vi "Perspective Calibration.vi"() -> ()   [LabVIEW 2014]
doc: "Description:\nThis example illustrates the use of a calibration grid to calibrate an image for perspective distortion and converts the locations of features found in the image into the locations in the real world. The example then performs accurate measurements in real world units using these locations.\n\nThis example loads a template image of a grid that is used to calibrate a system, uses the image loaded to learn the calibration from the grid, and measures distances of a distortion template with the learned calibration information."
uses:
  <vilib>/vision/Calibration.llb/Distortion Model.ctl
  <vilib>/vision/Calibration.llb/Distortion Model Types.ctl
  <vilib>/vision/Clamp.llb/Edge Polarity Type.ctl
  <vilib>/vision/Pattern Matching.llb/IMAQ Curve Parameters.ctl
  <vilib>/vision/NI_Vision_Development_Module.lvlib
panel:
  out "Clamp Results":T1(array[cluster])
  in  "Images Tab":T2(tab)
  out "Acquired Image":T3(plugin-control)
  out "Calibration Grid":T3(plugin-control)
  out "Segmented Holes":T3(plugin-control)
  out "Calibration Error Statistics":T4
  # "Overview: Demonstrates how to use a calibration grid to correct for perspective distortion and calculates the real world and pixel distances for parts to illustrate the importance of calibration to make accurate measurements. \nRequirements: Vision Development Software.\nInstructions: Run the VI."
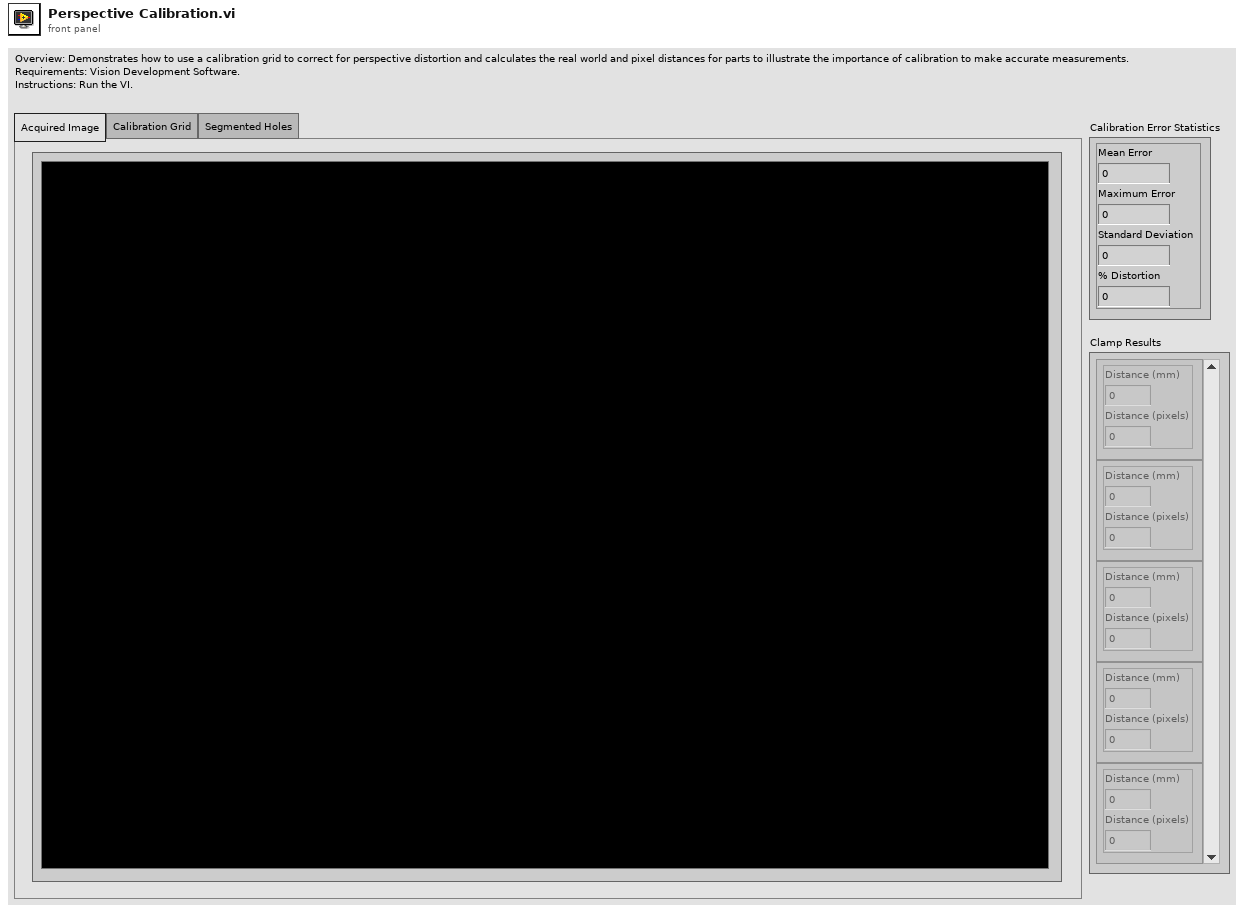
[diagram p1: front panel]
types:
  T1 = cluster{"Distance (mm)":dbl, "Distance (pixels)":dbl}[]
  T2 = enum32{"Acquired Image", "Calibration Grid", "Segmented Holes"}
  T3 = typedef "IMAQ Image.ctl" = refnum<image>
  T4 = cluster{"Mean Error":dbl, "Maximum Error":dbl, "Standard Deviation":dbl, "% Distortion":dbl}
  T5 = typedef "Distortion Model.ctl" = cluster{"Distortion Model":T6, "Polynomial Model Setup":cluster{"Radial Coefficient":u32, "Tangential Coefficients ":bool}}
  T6 = typedef "Distortion Model Types.ctl" = i32
  T7 = typedef "Particle Parameters" = i32
  T8 = cluster{"Measurement Parameter":T7, "Range Lower Value":dbl, "Range Upper Value":dbl, "Range":bool, "Measurement Type":bool}[]
  T9 = typedef "Image Unit" = enum32{"Undefined", "Angström", "Micrometer", "Millimeter", "Centimeter", "Meter", "Kilometer", "Microinch", "Inch", "Feet", "Nautical miles", "Standard miles", "Steps"}
  T10 = typedef "Calibration Reference Points.ctl" = cluster{"Pixel Coordinates":cluster{"X":dbl, "Y":dbl}[], "Real World Coordinates":cluster{"X":dbl, "Y":dbl}[], "Unit":T9, "Image Size":cluster{"X":u32, "Y":u32}}
  T11 = typedef "Error Statistics.ctl" = cluster{"Mean Error":dbl, "Maximum Error":dbl, "Standard Deviation":dbl, "% Distortion":dbl}
  T12 = cluster{"Area":dbl, "Number of Holes":dbl, "Bounding Rect":cluster{"Left":dbl, "Top":dbl, "Right":dbl, "Bottom":dbl}, "Center of Mass":cluster{"X":dbl, "Y":dbl}, "Orientation":dbl, "Dimensions":cluster{"Width":dbl, "Height":dbl}}[]
  T13 = typedef "IMAQ Curve Parameters.ctl" = cluster{"Extraction Mode":u32, "Edge Threshold":i32, "Edge Filter Size":u32, "Min Length":i32, "Row Search Step Size":i32, "Col Search Step Size":i32, "Max Endpoint Gap":i32, "Closed":bool, "Subpixel":bool}
  T14 = cluster{"Show Search Area":bool, "Show Curves":bool, "Show Clamp Locations":bool, "Show Result":bool, "Search Area Color":u32, "Curves Color":u32, "Clamp Locations Color":u32, "Result Color":u32, "Overlay Group Name":string}
  T15 = typedef "Edge Polarity Type.ctl" = u32
  T16 = cluster{"Angle Range (+/-)":dbl, "Edge Polarity":cluster{"Start":T15, "End":T15}}
  T17 = typedef "ROI Descriptor" = cluster{"Global Rectangle":i32[], "Contours":cluster{"ID":enum32{"External", "Internal"}, "Type":u32, "Coordinates":i32[]}[]}
  T18 = cluster{"Distance (Pixels)":dbl, "Distance (Real World)":dbl, "Angle (Absolute)":dbl, "Angle (Relative)":dbl}
  T19 = cluster{"Distance (Real World)":dbl, "Distance (Pixels)":dbl}
  T20 = cluster{"Distance (Real World)":dbl, "Distance (Pixels)":dbl}[]
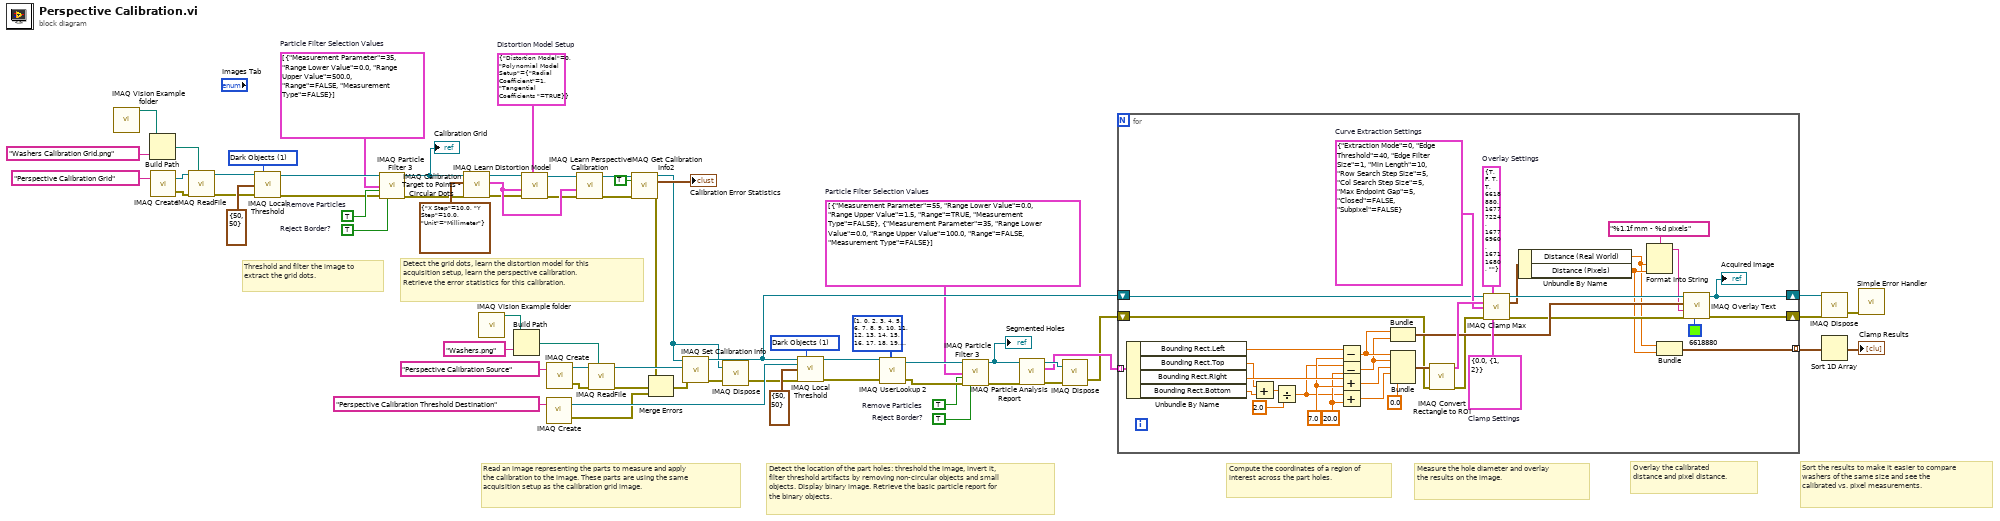
[diagram p0: block diagram]
diagram:
  w28 = TRUE  # Remove Particles
  w29 = TRUE  # Reject Border?
  w39 = T5 {"Distortion Model"=0, "Polynomial Model Setup"={"Radial Coefficient"=1, "Tangential Coefficients "=TRUE}}  # Distortion Model Setup
  w40 = T8 [{"Measurement Parameter"=35, "Range Lower Value"=0.0, "Range Upper Value"=500.0, "Range"=FALSE, "Measurement Type"=FALSE}]  # Particle Filter Selection Values
  w43 = TRUE  # Remove Particles
  w42 = TRUE  # Reject Border?
  w51 = u32 1 items=["Bright Objects", "Dark Objects"] ("Look For (Bright Objects)")
  w53 = T8 [{"Measurement Parameter"=55, "Range Lower Value"=0.0, "Range Upper Value"=1.5, "Range"=TRUE, "Measurement Type"=FALSE}, {"Measurement Parameter"=35, "Range Lower Value"=0.0, "Range Upper Value"=100.0, "Range"=FALSE, "Measurement Type"=FALSE}]  # Particle Filter Selection Values
  w60 = u32 1 items=["Bright Objects", "Dark Objects"] ("Look For (Bright Objects)")
  # "Sort the results to make it easier to compare washers of the same size and see the calibrated vs. pixel measurements."
  # "Overlay the calibrated distance and pixel distance."
  # "Detect the location of the part holes: threshold the image, invert it, filter threshold artifacts by removing non-circular objects and small objects. Display binary image. Retrieve the basic particle report for the binary objects."
  # "Measure the hole diameter and overlay the results on the image."
  # "Compute the coordinates of a region of interest across the part holes."
  # "Read an image representing the parts to measure and apply the calibration to the image. These parts are using the same acquisition setup as the calibration grid image."
  # "Detect the grid dots, learn the distortion model for this acquisition setup, learn the perspective calibration. Retrieve the error statistics for this calibration."
  # "Threshold and filter the image to extract the grid dots."
  n1 = call "IMAQ Vision Example folder.vi"() -> ("Example Image Path"=w26:path)  [unwired: 11 in]
  n2 = Build Path(base path=w26, name or relative path="Washers Calibration Grid.png") -> (appended path=w25:path)
  n3 = call "IMAQ Create"("Image Name"="Perspective Calibration Grid") -> ("New Image"=w64:T3, "error out"=w18:errorcluster)  [unwired: 3 in, 1 out]
  n4 = call "IMAQ ReadFile"("File Path"=w25, "error in (no error)"=w18, "Image"=w64) -> ("error out"=w38:errorcluster, "Image Out"=w21:T3)  [unwired: 2 in, 5 out]
  n5 = call "IMAQ Local Threshold"("Image Src"=w21, "Look For (Bright Objects)"=w51, "Window Size (32x32)"=cluster{"SizeX":i32, "SizeY":i32} {"SizeX"=50, "SizeY"=50}, "error in (no error)"=w38) -> ("Image Dst Out"=w41:T3, "error out"=w37:errorcluster)  [unwired: 4 in, 6 out]
  n6 = call "IMAQ Particle Filter 3"("Image Src"=w41, "Selection Values"=w40, "Keep/Remove Particles (F)"=w43, "error in (no error)"=w37, "Reject Border? (F)"=w42) -> ("Image Dst Out"=w20:T3, "error out"=w36:errorcluster)  [unwired: 4 in, 5 out]
  "Calibration Grid" <- w20
  n7 = call "IMAQ Calibration Target to Points - Circular Dots"("error in (no error)"=w36, "Grid Descriptor"=cluster{"X Step":sgl, "Y Step":sgl, "Unit":T9} {"X Step"=10.0, "Y Step"=10.0, "Unit"=enum."Millimeter"}, "Target Image"=w20) -> ("error out"=w35:errorcluster, "Reference Points"=w48:T10, "Target Image (dup)"=w50:T3)  [unwired: 2 in, 4 out]
  n8 = call "IMAQ Vision Example folder.vi"() -> ("Example Image Path"=w24:path)  [unwired: 11 in]
  n9 = Build Path(base path=w24, name or relative path="Washers.png") -> (appended path=w22:path)
  n10 = call "IMAQ Learn Distortion Model"("Distortion Model Setup"=w39, "error in (no error)"=w35, "Reference Points"=w48, "Calibration Template Image"=w50) -> ("error out"=w34:errorcluster, "Calibration Template Image Out"=w49:T3)  [unwired: 2 in, 4 out]
  n11 = call "IMAQ Create"("Image Name"="Perspective Calibration Threshold Destination") -> ("New Image"=w61:T3, "error out"=w13:errorcluster)  [unwired: 3 in, 1 out]
  n12 = call "IMAQ Create"("Image Name"="Perspective Calibration Source") -> ("New Image"=w63:T3, "error out"=w17:errorcluster)  [unwired: 3 in, 1 out]
  n13 = call "IMAQ Learn Perspective Calibration"("error in (no error)"=w34, "Reference Points"=w48, "Calibration Template Image"=w49) -> ("error out"=w33:errorcluster, "Calibration Template Image Out"=w47:T3)  [unwired: 1 in, 6 out]
  n14 = call "IMAQ ReadFile"("File Path"=w22, "error in (no error)"=w17, "Image"=w63) -> ("error out"=w16:errorcluster, "Image Out"=w56:T3)  [unwired: 2 in, 5 out]
  n15 = call "IMAQ Get Calibration Info2"("Calibration Template Image"=w47, "Return Error Information (False)"=TRUE, "error in (no error)"=w33) -> ("Calibration Template Image (duplicate)"=w3:T3, "Error Statistics"=→"Calibration Error Statistics":T11, "error out"=w15:errorcluster)  [unwired: 10 out]
  n16 = Merge Errors(w15, w16, w13) -> (w14:errorcluster)
  n17 = call "IMAQ Set Calibration Info"("error in (no error)"=w14, "Image Dst"=w56, "Image Src"=w3) -> ("error out"=w4:errorcluster, "Calibrated Image"=w57:T3)  [unwired: 1 in, 6 out]
  n18 = call "IMAQ Dispose"("Image"=w3, "error in (no error)"=w4) -> ("error out"=w2:errorcluster)  [unwired: 4 in]
  n19 = call "IMAQ Local Threshold"("Image Src"=w57, "Look For (Bright Objects)"=w60, "Image Dst"=w61, "Window Size (32x32)"=cluster{"SizeX":i32, "SizeY":i32} {"SizeX"=50, "SizeY"=50}, "error in (no error)"=w2) -> ("Image Dst Out"=w58:T3, "error out"=w32:errorcluster)  [unwired: 3 in, 6 out]
  n20 = call "IMAQ UserLookup 2"("Image Src"=w58, "Lookup Table"=i32[] [1, 0, 2, 3, 4, 5, 6, 7, 8, 9, 10, 11, 12, 13, 14, 15, 16, 17, 18, 19, 20, 21, 22, 23, 24, 25, 26, 27, 28, 29, 30, 31, 32, 33, 34, 35, 36, 37, 38, 39, 40, 41, 42, 43, 44, 45, 46, 47, 48, 49, 50, 51, 52, 53, 54, 55, 56, 57, 58, 59, 60, 61, 62, 63, 64, 65, 66, 67, 68, 69, 70, 71, 72, 73, 74, 75, 76, 77, 78, 79, 80, 81, 82, 83, 84, 85, 86, 87, 88, 89, 90, 91, 92, 93, 94, 95, 96, 97, 98, 99, 100, 101, 102, 103, 104, 105, 106, 107, 108, 109, 110, 111, 112, 113, 114, 115, 116, 117, 118, 119, 120, 121, 122, 123, 124, 125, 126, 127, 128, 129, 130, 131, 132, 133, 134, 135, 136, 137, 138, 139, 140, 141, 142, 143, 144, 145, 146, 147, 148, 149, 150, 151, 152, 153, 154, 155, 156, 157, 158, 159, 160, 161, 162, 163, 164, 165, 166, 167, 168, 169, 170, 171, 172, 173, 174, 175, 176, 177, 178, 179, 180, 181, 182, 183, 184, 185, 186, 187, 188, 189, 190, 191, 192, 193, 194, 195, 196, 197, 198, 199, 200, 201, 202, 203, 204, 205, 206, 207, 208, 209, 210, 211, 212, 213, 214, 215, 216, 217, 218, 219, 220, 221, 222, 223, 224, 225, 226, 227, 228, 229, 230, 231, 232, 233, 234, 235, 236, 237, 238, 239, 240, 241, 242, 243, 244, 245, 246, 247, 248, 249, 250, 251, 252, 253, 254, 255], "error in (no error)"=w32) -> ("Image Dst Out"=w54:T3, "error out"=w31:errorcluster)  [unwired: 2 in, 2 out]
  n21 = call "IMAQ Particle Filter 3"("Image Src"=w54, "Selection Values"=w53, "Keep/Remove Particles (F)"=w28, "error in (no error)"=w31, "Reject Border? (F)"=w29) -> ("Image Dst Out"=w19:T3, "error out"=w30:errorcluster)  [unwired: 4 in, 5 out]
  "Segmented Holes" <- w19
  n22 = call "IMAQ Particle Analysis Report"("error in (no error)"=w30, "Image"=w19) -> ("error out"=w12:errorcluster, "Particle Reports (Pixels)"=w10:T12, "Image Out (duplicate)"=w11:T3)  [unwired: 1 in, 6 out]
  n23 = call "IMAQ Dispose"("Image"=w11, "error in (no error)"=w12) -> ("error out"=w9:errorcluster)  [unwired: 4 in]
  n24 = for {
    tunnel: w10 -> [w101] mode=indexing
    shift-right: [w72] -> w7
    shift-left: w57 -> [w83]
    shift-right: [w74] -> w8
    shift-left: w9 -> [w68]
    tunnel: [w69] -> w6 mode=indexing
    w90 = T13 {"Extraction Mode"=0, "Edge Threshold"=40, "Edge Filter Size"=1, "Min Length"=10, "Row Search Step Size"=5, "Col Search Step Size"=5, "Max Endpoint Gap"=5, "Closed"=FALSE, "Subpixel"=FALSE}  # Curve Extraction Settings
    w88 = T14 {"Show Search Area"=TRUE, "Show Curves"=FALSE, "Show Clamp Locations"=TRUE, "Show Result"=TRUE, "Search Area Color"=6618880, "Curves Color"=16777224, "Clamp Locations Color"=16776960, "Result Color"=16711680, "Overlay Group Name"=""}  # Overlay Settings
    w89 = T16 {"Angle Range (+/-)"=0.0, "Edge Polarity"={"Start"=1, "End"=2}}  # Clamp Settings
    w93 = 20.0 ("y")
    w98 = 7.0 ("y")
    n25 = Unbundle By Name(w101) -> ("Bounding Rect.Left"=w86:dbl, "Bounding Rect.Top"=w77:dbl, "Bounding Rect.Right"=w99:dbl, "Bounding Rect.Bottom"=w76:dbl)
    n26 = Add(x=w77, y=w76) -> (x+y=w95:dbl)
    n27 = Divide(x=w95, y=2.0) -> (x/y=w84:dbl)
    n28 = Subtract(x=w86, y=w98) -> (x-y=w81:dbl)
    n29 = Subtract(x=w84, y=w93) -> (x-y=w80:dbl)
    n30 = Add(x=w99, y=w98) -> (x+y=w97:dbl)
    n31 = Add(x=w84, y=w93) -> (x+y=w96:dbl)
    n32 = Bundle(w81, w80) -> (w79:cluster{dbl, dbl})  [unwired: 1 out]
    n33 = Bundle(w81, w80, w97, w96, "y"=0.0) -> (w100:cluster{dbl, dbl, dbl, dbl, "y":dbl})  [unwired: 1 out]
    n34 = call "IMAQ Convert Rectangle to ROI"("error in (no error)"=w68, "Rectangle"=w100) -> ("error out"=w67:errorcluster, "ROI Descriptor"=w91:T17)  [unwired: 7 out]
    n35 = call "IMAQ Clamp Max"("Source Image"=w83, "Overlay Settings"=w88, "ROI Descriptor"=w91, "Curve Extraction Settings"=w90, "error in (no error)"=w67, "Clamp Settings"=w89) -> ("Image Out"=w82:T3, "Clamp Results"=w75:T18, "error out"=w73:errorcluster)  [unwired: 1 in, 6 out]
    n36 = Unbundle By Name(w75) -> ("Distance (Real World)"=w70:dbl, "Distance (Pixels)"=w71:dbl)
    n37 = Format Into String(format string="%1.1f mm - %d pixels", w70, w71) -> (resulting string=w78:string)  [unwired: 2 in, 1 out]
    n38 = Bundle("Distance (Real World)"=w70, "Distance (Pixels)"=w71) -> (w69:T19)  [unwired: 1 in]
    n39 = call "IMAQ Overlay Text"("Text Color (black)"=u32 6618880, "error in (no error)"=w73, "String"=w78, "Origin"=w79, "Image"=w82) -> ("error out"=w74:errorcluster, "Image Out"=w72:T3)  [unwired: 3 in, 2 out]
    "Acquired Image" <- w72
  }
  n40 = call "IMAQ Dispose"("Image"=w7, "error in (no error)"=w8) -> ("error out"=w1:errorcluster)  [unwired: 4 in]
  n41 = Sort 1D Array(array=w6) -> (sorted array=→"Clamp Results":T20)
  n42 = call <vilib>:"Simple Error Handler.vi"("error in (no error)"=w1) -> ()  [unwired: 1 in, 8 out]
